vi "Flush qeueu worker.vi"(8 "error in (no error)":errorcluster, 11 "gRPC Client in":refnum<class "gRPC Client.lvclass">) -> (0 "error out":errorcluster, 3 "reference out":refnum<class "gRPC Client.lvclass">)   [LabVIEW 2023, in "gRPC Client.lvclass"]
uses:
  gRPC Client.lvclass
  gRPC Client.lvclass/gRPC Client.ctl
  <vilib>/addons/_Workers/Library/Classes/Message Queue/Message Queue.lvclass
panel:
  # "Connector Pane"
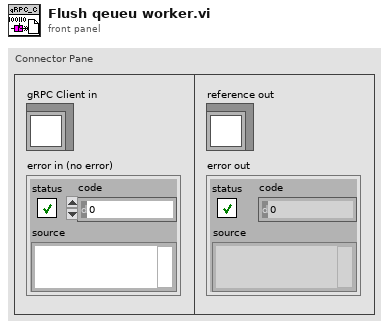
[diagram p1: front panel]
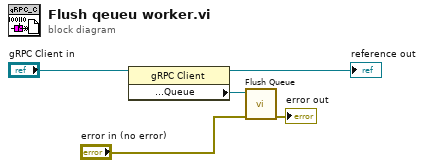
[diagram p0: block diagram]
diagram:
  n1 = property class="gRPC Client"(reference="gRPC Client in") -> (reference out=→"reference out":refnum<class "gRPC Client.lvclass">, "Accessors:Read:Public API:Queue"=w5:refnum<class "Message Queue.lvclass">)  [unwired: 1 in, 1 out]
  n2 = call <vilib>:"Flush Queue.vi"("error in (no error)"="error in (no error)", "Message Queue"=w5) -> ("error out"=→"error out":errorcluster)  [unwired: 7 in, 2 out]
